vi "Global_CalibrationSimulation.vi"() -> ()   [LabVIEW 2012]
panel:
  in  "Galvo Uncage Path":path=path "D:/Dual Channel Test Images - SciScan/2016_09_20/20160920_11_10_37_galvo_uncage_green_800nm/20160920_11_10_37_galvo_uncage_green_800nm_XYT_ch_1.bmp"
  in  "Reso Image Path":path=path "D:/Dual Channel Test Images - SciScan/2016_09_20/20160920_10_45_54_resonant_800nm_green/20160920_10_45_54_resonant_800nm_green_XYT_ch_1.bmp"
  in  "Galvo Image Path":path=path "D:/Dual Channel Test Images - SciScan/2016_09_20/20160920_11_04_00_galvo_image_green_800nm/20160920_11_04_00_galvo_image_green_800nm_XYT_ch_1.bmp"
  in  "Simulation?":bool
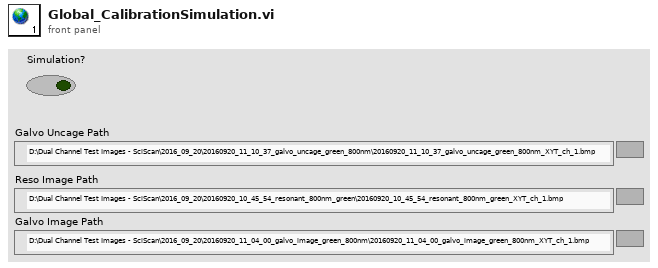
[diagram p1: front panel]
diagram:
